vi "change control.vi"(8 "error in (no error)":errorcluster, 10 "type definition":T1, 11 "Control in":refnum<vi>) -> (0 "error out":errorcluster, 3 "control out":refnum<vi>)   [LabVIEW 2013] (continued)
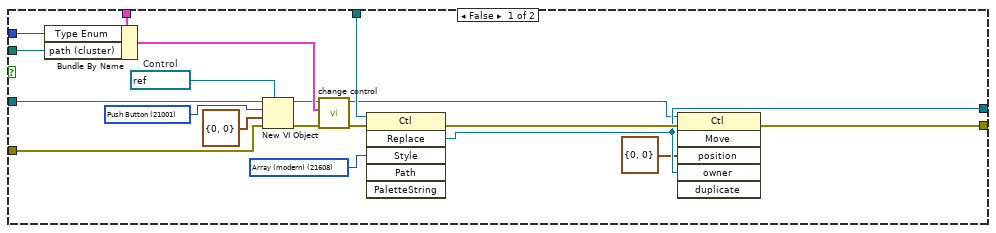
[diagram p16: hidden frame]
